vi "add_tcp_connection.vi"(4 "error in":errorcluster, 7 "Sensor connection":refnum<k5>) -> (0 "error out":errorcluster)   [LabVIEW 2019, in "Lib_Simx.lvlib"]
doc: "Add a TCP reference to the simx global varible."
uses:
  Lib_Simx.lvlib
  tools/simx_common.vi
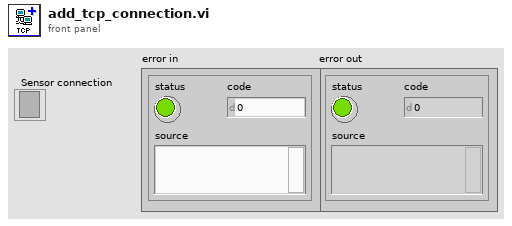
[diagram p1: front panel]
types:
  T1 = typedef "Lib_Simx.lvlib/simx_connection.ctl" = cluster{"Config":T2, "Connections":T5, "Map":cluster{"lanes":cluster{"x":dbl[], "y":dbl[], "z":dbl[]}, "StartPosition":cluster{"start_points":T6, "StartRotation":dbl[], "StartLocation":dbl[]}, "Draw Map Size":T7, "DrawArea":cluster{"min_Y":dbl, "min_X":dbl, "Scale X":dbl, "Scale Y":dbl}, "Map":picture, "Map Geojson":string}}
  T2 = typedef "Lib_Simx.lvlib/config.ctl" = cluster{"Trajectory":T3, "Weather":T4}
  T3 = typedef "Lib_Simx.lvlib/trajectory.ctl" = cluster{"Number of frames":i32, "Frame number":i32, "Trajectory":string}
  T4 = typedef "Lib_Simx.lvlib/weather.ctl" = cluster{"id":string}
  T5 = typedef "Lib_Simx.lvlib/connections.ctl" = cluster{"Simulator Connection":refnum<k5>, "server_ip":string, "Port":i32, "Sensor connections":refnum<k5>[]}
  T6 = typedef "Lib_Simx.lvlib/start_points.ctl" = cluster{"locations":dbl[][], "rotations":dbl[][], "type":string[]}
  T7 = typedef "LVBoundsTypeDef.ctl" = cluster{"Width":u32, "Height":u32}
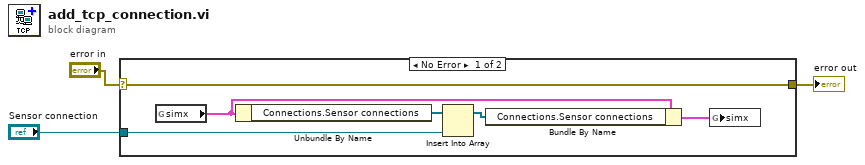
[diagram p0: block diagram]
diagram:
  n1 = case shown="No Error" "error in" {
    selector: "error in" -> [w4 w10]
    tunnel: "Sensor connection" -> [w5 _]
    tunnel: [w4 w10] -> w1
    frame No Error {
      n2 = global read "simx_common.vi" "simx"() -> (w7:T1)
      n3 = Unbundle By Name(w7) -> ("Connections.Sensor connections"=w8:refnum<k5>[])
      n4 = Insert Into Array(array=w8, new element=w5) -> (w9:refnum<k5>[])  [unwired: 1 in]
      n5 = Bundle By Name(cluster=w7, "Connections.Sensor connections"=w9) -> (w6:T1)
      n6 = global write "simx_common.vi" "simx"(w6) -> ()
    }
    frame Error {
    }
  }
  "error out" <- w1
